vi "_Read.vi"(8 "error in (no error)":errorcluster, 10 "Count":i32, 11 "WebsocketStream in":refnum<class "WebsocketStream.lvclass">) -> (0 "error out":errorcluster, 2 "Data":string, 3 "WebsocketStream out":refnum<class "WebsocketStream.lvclass">)   [LabVIEW 2020, in "Stream-Websocket.lvlib" / "WebsocketStream.lvclass"]
uses:
  WebsocketStream.lvclass
  WebsocketStream.lvclass/WebsocketStream.ctl
  Lock Type.ctl
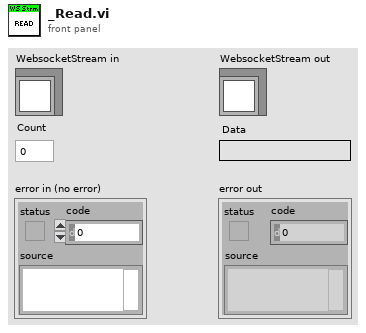
[diagram p1: front panel]
types:
  T1 = typedef "Stream-Websocket.lvlib/WebsocketStream.lvclass/Lock Type.ctl" = enum16{"Read", "Write"}
  T2 = typedef "Stream-Websocket.lvlib/Message Frame.ctl" = cluster{"FIN":bool, "RSV1":bool, "RSV2":bool, "RSV3":bool, "MASK":bool, "OpCode":T3, "Length":u64, "MaskingKey":u8[], "Payload":string}
  T3 = typedef "Stream-Websocket.lvlib/OpCode.ctl" = enum8{"Continuation", "Text", "Binary", "Reserved3", "Reserved4", "Reserved5", "Reserved6", "Reserved7", "Close", "Ping", "Pong", "ReservedB", "ReservedC", "ReservedD", "ReservedE", "ReservedF"}
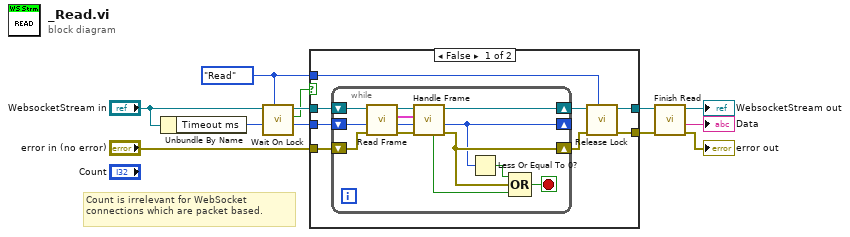
[diagram p0: block diagram]
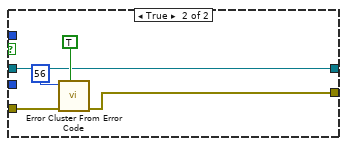
[diagram p2: hidden frame]
diagram:
  w1 = Lock_Type."Read" ("Lock Type")
  # "Count is irrelevant for WebSocket connections which are packet based."
  n1 = Unbundle By Name("WebsocketStream in") -> ("Timeout ms"=w5:i32)
  n2 = call "Wait On Lock.vi"("Lock Type"=w1, "Timeout ms"=w5, "WebsocketStream in"="WebsocketStream in") -> ("Remaining  Timeout"=w6:i32, "Timeout"=w3:bool, "WebsocketStream out"=w7:refnum<class "WebsocketStream.lvclass">)  [unwired: 5 in, 1 out]
  n3 = case shown="False" w3 {
    tunnel: [w16 w34] -> w2
    tunnel: [w14 w35] -> w10
    tunnel: w7 -> [w20 w34]
    tunnel: w6 -> [w19 _]
    tunnel: "error in (no error)" -> [w18 w38]
    tunnel: w1 -> [w13 _]
    frame False {
      n4 = while {
        shift-right: [w21] -> w17
        shift-left: w20 -> [w32]
        shift-right: [w33] -> w15
        shift-left: w18 -> [w31]
        shift-right: [w24] -> _
        shift-left: w19 -> [w30]
        stop <- w29 stop-if-true
        n5 = call "Read Frame.vi"("error in (no error)"=w31, "Timeout ms"=w30, "WebsocketStream in"=w32) -> ("error out"=w25:errorcluster, "Remaining  Timeout"=w26:i32, "Frame"=w27:T2, "WebsocketStream out"=w28:refnum<class "WebsocketStream.lvclass">)  [unwired: 5 in]
        n6 = call "Handle Frame.vi"("error in (no error)"=w25, "Timeout ms"=w26, "Frame In"=w27, "WebsocketStream in"=w28) -> ("error out"=w33:errorcluster, "Remaining  Timeout"=w24:i32, "WebsocketStream out"=w21:refnum<class "WebsocketStream.lvclass">, "Done?"=w23:bool)  [unwired: 4 in]
        n7 = Less Or Equal To 0?(x=w24) -> (x <= 0?=w22:bool)
        n8 = Compound Arithmetic op=OR(w22, w33, w23) -> (w29:bool)
      }
      n9 = call "Release Lock.vi"("Lock Type"=w13, "error in (no error)"=w15, "WebsocketStream in"=w17) -> ("error out"=w14:errorcluster, "WebsocketStream out"=w16:refnum<class "WebsocketStream.lvclass">)  [unwired: 7 in]
    }
    frame True {
      n10 = call <vilib>:"Error Cluster From Error Code.vi"("show call chain? (False)"=TRUE, "error in (no error)"=w38, "error code (0)"=56) -> ("error out"=w35:errorcluster)  [unwired: 6 in]
    }
  }
  n11 = call "Finish Read.vi"("error in (no error)"=w10, "WebsocketStream in"=w2) -> ("error out"=→"error out":errorcluster, "Data"=→"Data":string, "WebsocketStream out"=→"WebsocketStream out":refnum<class "WebsocketStream.lvclass">)  [unwired: 7 in]
